vi "test query_components.vi"() -> ()   [LabVIEW 2023]
uses:
  DB Component.ctl
  Database.lvlib
panel:
  in  "version":i32=1
  in  "part":string
  out "Components":T1[](array[typedef])
  out "error out":errorcluster
  in  "port":i32=33060
  in  "host":string="localhost"
  in  "password":string="carriker"
  in  "username":string="root"
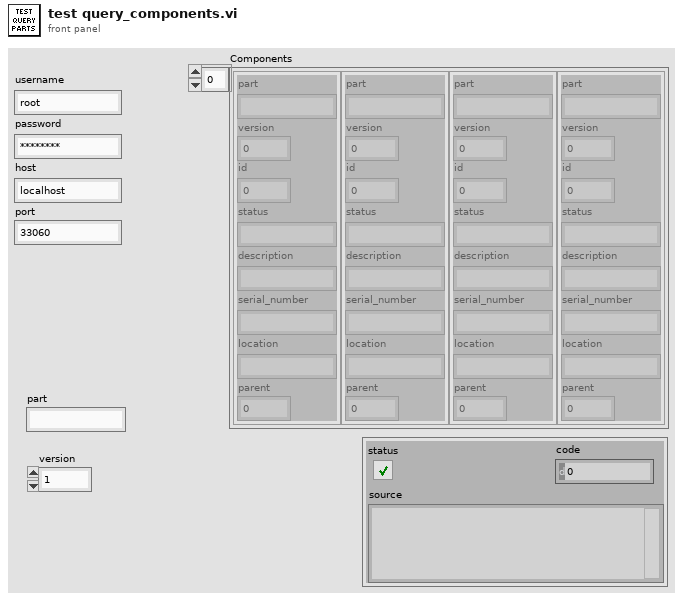
[diagram p1: front panel]
types:
  T1 = typedef "Database.lvlib/DB Component.ctl" = cluster{"part":string, "version":i32, "id":i32, "status":string, "description":string, "serial_number":string, "location":string, "parent":i32}
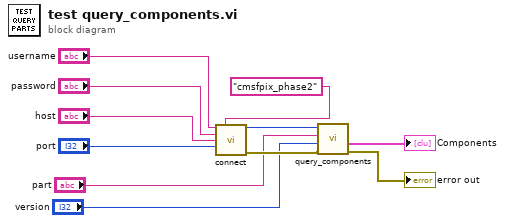
[diagram p0: block diagram]
diagram:
  n1 = call "connect.vi"("username"="username", "schema"="cmsfpix_phase2" ("Schema"), "password"="password", "host"="host", "port"="port") -> ("DB Session ID"=w7:i32, "error out"=w6:errorcluster)  [unwired: 9 in]
  n2 = call "query_components.vi"("error in (no error)"=w6, "version"="version", "part"="part", "DB Session ID"=w7) -> ("error out"=→"error out":errorcluster, "Components"=→"Components":T1[])  [unwired: 5 in, 1 out]
